vi "LINX - PmodGPS.vi"() -> ()   [LabVIEW 2019]
doc: "PmodGPS\n\nThis example demonstrates how to read GPS information from PmodGPS.\n\nInstructions:\n1. Select the COM Port associated with the LINX device\n2. Select the UART Channel that the Pmod is connected to.\n3. Click the Run Arrow."
uses:
  <vilib>/MakerHub/LINX/Public/Utilities/Open Serial.vi
  <vilib>/MakerHub/LINX/Public/Sensors/Pmods/GPS/PmodGPS.lvlib
  <vilib>/MakerHub/LINX/LMH-LINX.lvlib
panel:
  out "Output Cluster":T1
  in  "Serial Port":refnum<visa-resource-name>="N/A"
  in  "UART Channel (0)":u8
  in  "Stop Button":bool
  # "PmodGPS\n\nThis example demonstrates how to read GPS information from PmodGPS.\n\nInstructions:\n1. Select the COM Port associated with the LINX device\n2. Select the UART Channel that the Pmod is connected to.\n3. Click the Run Arrow."
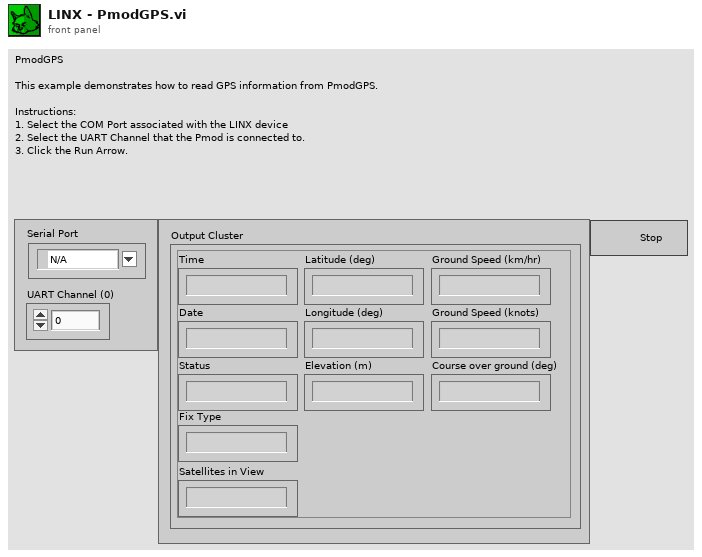
[diagram p1: front panel]
types:
  T1 = cluster{"Time":string, "Date":string, "Status":string, "Fix Type":string, "Satellites in View":string, "Latitude (deg)":string, "Longitude (deg)":string, "Elevation (m)":string, "Ground Speed (km/hr)":string, "Ground Speed (knots)":string, "Course over ground (deg)":string}
  T2 = typedef "LMH-LINX.lvlib/LINX Ref.ctl" = cluster{"IO":T3, "Interface":T4, "LINX Device Config":T5}
  T3 = typedef "LMH-LINX.lvlib/Platform.ctl" = enum16{"Remote", "Local"}
  T4 = typedef "LMH-LINX.lvlib/Interface.ctl" = enum16{"Serial", "TCP"}
  T5 = typedef "LMH-LINX.lvlib/Device.lvlib/LINX Device Config.ctl" = cluster{"Interface":T4, "COM Port":refnum<visa-resource-name>, "TCP Configuration":T6, "Device Family":u8, "Device ID":u8, "Device Name":string, "TCP Ref":refnum<k5>, "Channels":T7}
  T6 = typedef "LMH-LINX.lvlib/Device.lvlib/TCP Config.ctl" = cluster{"IP Address":string, "Port":u16}
  T7 = typedef "LMH-LINX.lvlib/Channels.ctl" = cluster{"DI":u8[], "DO":u8[], "AI":u8[], "AO":u8[], "PWM":u8[], "QE":u8[], "UART":u8[], "I2C 2":u8[], "SPI":u8[], "CAN":u8[], "Servo":u8[], "AI Ref (V)":dbl, "AI Resolution (Bits)":u8, "AO Ref (V)":dbl, "AO Resolution (Bits)":u8}
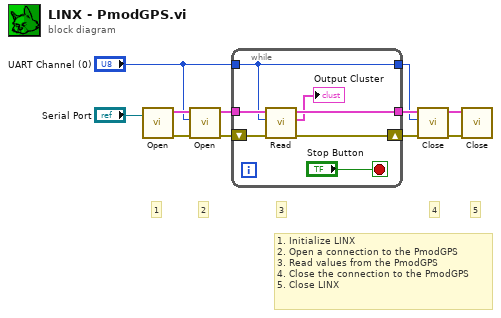
[diagram p0: block diagram]
diagram:
  # "1. Initialize LINX\n2. Open a connection to the PmodGPS\n3. Read values from the PmodGPS\n4. Close the connection to the PmodGPS\n5. Close LINX"
  # "5"
  # "4"
  # "3"
  # "2"
  # "1"
  n1 = call-poly <vilib>:"Open.vi"("Serial Port"="Serial Port") -> ("Error Out"=w7:errorcluster, "LINX Resource"=w6:T2)  [unwired: 8 in, 1 out]
  n2 = call <vilib>:"Open.vi"("Error In"=w7, "UART Channel (0)"="UART Channel (0)", "LINX Ref"=w6) -> ("Error Out"=w11:errorcluster, "LINX Resource"=w10:T2)  [unwired: 7 in]
  n3 = while {
    tunnel: w10 -> [w16]
    tunnel: [w15] -> w9
    shift-right: [w14] -> w8
    shift-left: w11 -> [w17]
    tunnel: "UART Channel (0)" -> [w12]
    tunnel: [w12] -> w1
    stop <- "Stop Button" stop-if-true
    n4 = call <vilib>:"Read.vi"("Error In"=w17, "UART Channel (0)"=w12, "LINX Resource"=w16) -> ("Error Out"=w14:errorcluster, "GPS Data"=→"Output Cluster":T1, "LINX Resource"=w15:T2)  [unwired: 6 in]
  }
  n5 = call <vilib>:"Close.vi"("error in (no error)"=w8, "UART Channel (0)"=w1, "LINX Resource"=w9) -> ("error out"=w2:errorcluster, "LINX Resource out"=w3:T2)  [unwired: 7 in]
  n6 = call <vilib>:"Close.vi"("Error In"=w2, "LINX Resource"=w3) -> ()  [unwired: 9 in, 1 out]
